vi "Init Tunnel References.vi"(8 "error in (no error)":errorcluster, 11 "CSM-Helper in":refnum<class "CSM-Helper.lvclass">) -> (0 "error out":errorcluster, 3 "CSM-Helper out":refnum<class "CSM-Helper.lvclass">)   [LabVIEW 2020, in "CSM-Helper.lvclass"]
uses:
  CSM-Helper.lvclass
  CSM-Helper.lvclass/CSM-Helper.ctl
  <vilib>/Utility/Data Type/Type Definitions/Data Type.ctl
  <vilib>/Utility/Data Type/Type Definitions/Refnum Type.ctl
  <vilib>/Utility/Data Type/NI_Data Type.lvlib
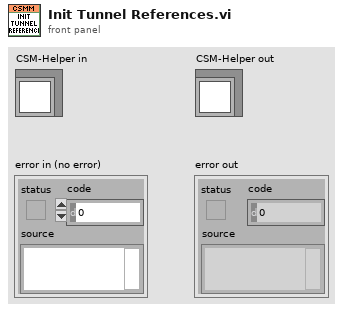
[diagram p1: front panel]
types:
  T1 = cluster{refnum<vi>, "Outer Term":refnum<vi>, "Data Type":variant, "Wire":refnum<vi>}
  T2 = typedef "NI_Data Type.lvlib/Data Type.ctl" = enum8{"Invalid Type", "Void", "I8", "I16", "I32", "I64", "U8", "U16", "U32", "U64", "Single Float", "Double Float", "Extended Float", "Single Complex", "Double Complex", "Extended Complex", "Enum U8", "Enum U16", "Enum U32", "Enum U64", "Single Float With Unit", "Double Float With Unit", "Extended Float With Unit", "Single Complex with Unit", "Double Complex with Unit", "Extended Complex with Unit", "Boolean", "String", "Path", "Picture", "Tag", "Array", "Cluster", "Variant", "LV Variant", "Waveform", "Timestamp", "Digital Waveform", "Digital Data", "ExpressData", "Refnum", "External Data", "VI", "Poly VI", "LabVIEW Class Instance", "Fixed Point", "Set Collection", "Map Collection"}
  T3 = typedef "NI_Data Type.lvlib/Type Definition Info.ctl" = cluster{"Name":string, "Timestamp":u32}
  T4 = typedef "NI_Data Type.lvlib/Refnum Type.ctl" = enum16{"NotARefnum", "UnknownRefnum", "Generic", "Datalog", "ByteStream", "Device", "Occurence", "TCPNetConnection", "Auto", "Menu", "Imaq", "Hardware", "DataSocket", "Visa", "IVI", "UDPNetConnection", "Notifier", "Queue", "Irda", "EventReg", "DotNet", "UserEvent", "Callback", "UNUSED_EMPTY_POSITION", "BlueToothNetConnection", "LVObjApp", "LVObjVI", "LVObjUnknown", "GenericClass", "UserDefinedRefnumTag", "DataValue", "RT FIFO", "TDMS File", "PythonSessionRefnum"}
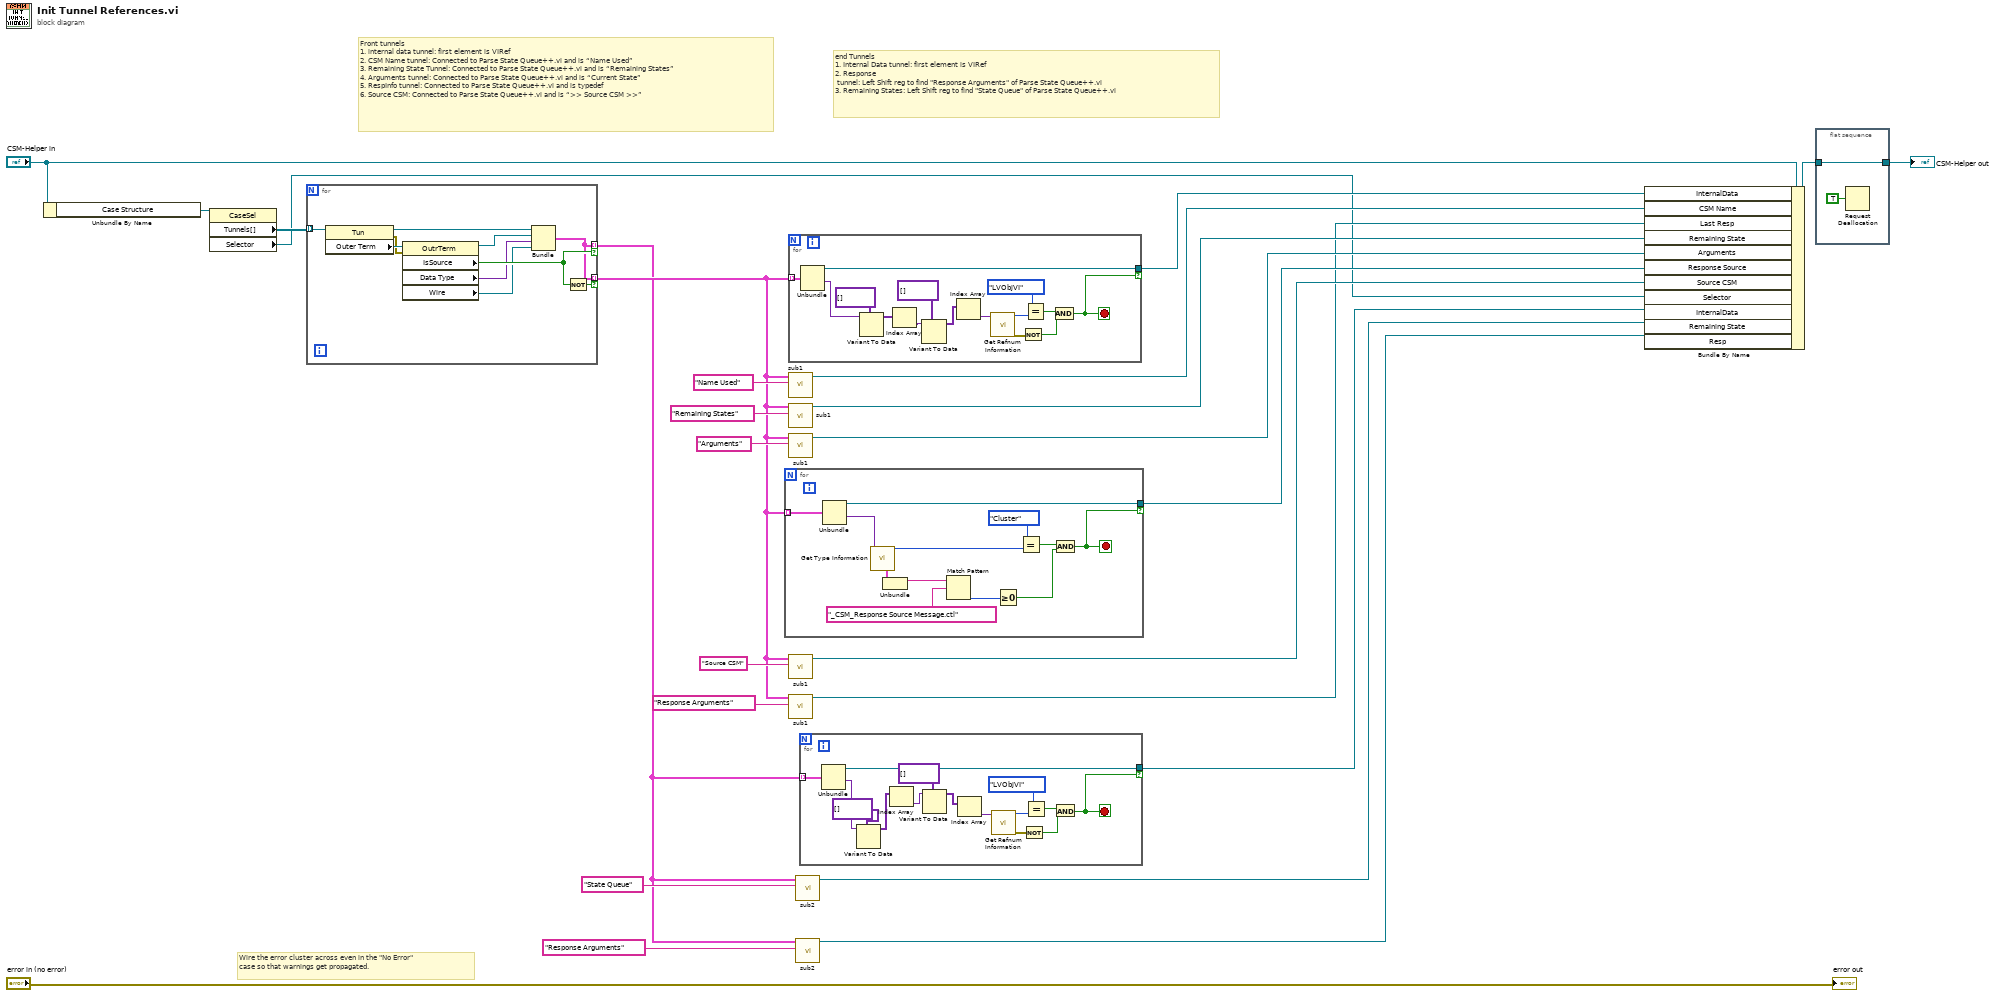
[diagram p0: block diagram]
diagram:
  # "end Tunnels\n1. Internal Data tunnel: first element is VIRef\n2. Response\n tunnel: Left Shift reg to find \"Response Arguments\" of Parse State Queue++.vi \n3. Remaining States: Left Shift reg to find \"State Queue\" of Parse State Queue++.vi"
  # "Front tunnels\n1. internal data tunnel: first element is VIRef\n2. CSM Name tunnel: Connected to Parse State Queue++.vi and is “Name Used”\n3. Remaining State Tunnel: Connected to Parse State Queue++.vi and is “Remaining States”\n4. Arguments tunnel: Connected to Parse State Queue++.vi and is “Current State”\n5. RespInfo tunnel: Connected to Parse State Queue++.vi and is typedef\n6. Source CSM: Connected to Parse State Queue++.vi and is “>> Source CSM >>”"
  # "Wire the error cluster across even in the \"No Error\"\ncase so that warnings get propagated."
  n1 = Unbundle By Name("CSM-Helper in") -> ("Case Structure"=w24:refnum<vi>)
  n2 = property class="CaseSel"(reference=w24) -> ("Tunnels[]"=w23:refnum<vi>[], "Selector"=w9:refnum<vi>)  [unwired: 1 in, 2 out]
  n3 = for {
    tunnel: w23 -> [w36] mode=indexing
    tunnel: [w29] -> w3 mode=indexing if=w33
    tunnel: [w29] -> w12 mode=indexing if=w32
    n4 = property class="Tun"(reference=w36) -> (reference out=w31:refnum<vi>, error out=w34:errorcluster, "Outer Term"=w35:refnum<vi>)  [unwired: 1 in]
    n5 = property class="OutrTerm"(reference=w35, error in=w34) -> (reference out=w30:refnum<vi>, "IsSource"=w33:bool, "Data Type"=w28:variant, "Wire"=w27:refnum<vi>)  [unwired: 1 out]
    n6 = Bundle(w31, "Outer Term"=w30, "Data Type"=w28, "Wire"=w27) -> (w29:T1)  [unwired: 1 in]
    n7 = Not(x=w33) -> (.not. x?=w32:bool)
  }
  n8 = for {
    tunnel: w12 -> [w48] mode=indexing
    tunnel: [w45] -> w13 if=w44
    stop <- w44 stop-if-true
    n9 = Unbundle(w48) -> (w45:refnum<vi>, "Data Type"=w41:variant)  [unwired: 2 out]
    n10 = call <vilib>:"Get Type Information.vi"("variant"=w41) -> ("type"=w47:T2, "type definition info"=w42:T3)  [unwired: 6 in, 3 out]
    n11 = Unbundle(w42) -> ("Name"=w40:string)  [unwired: 1 out]
    n12 = Match Pattern(string=w40, regular expression="_CSM_Response Source Message.ctl") -> (offset past match=w38:i32)  [unwired: 1 in, 3 out]
    n13 = Greater Or Equal To 0?(x=w38) -> (x >= 0?=w37:bool)
    n14 = Equal?(x=Data_Type."Cluster", y=w47) -> (x = y?=w46:bool)
    n15 = And(x=w46, y=w37) -> (x .and. y?=w44:bool)
  }
  n16 = for {
    tunnel: w12 -> [w63] mode=indexing
    tunnel: [w56] -> w22 if=w55
    stop <- w55 stop-if-true
    n17 = Unbundle(w63) -> (w56:refnum<vi>, "Data Type"=w53:variant)  [unwired: 2 out]
    n18 = Variant To Data(type=variant[] [] ("Array"), Variant=w53) -> (data=w52:variant[])  [unwired: 1 in, 1 out]
    n19 = Index Array(array=w52) -> (element=w50:variant)  [unwired: 1 in]
    n20 = Variant To Data(type=variant[] [] ("Array"), Variant=w50) -> (data=w49:variant[])  [unwired: 1 in, 1 out]
    n21 = Index Array(array=w49) -> (element=w62:variant)  [unwired: 1 in]
    n22 = call <vilib>:"Get Refnum Information.vi"("variant"=w62) -> ("error out"=w58:errorcluster, "reference type"=w60:T4)  [unwired: 7 in, 2 out]
    n23 = Not(x=w58) -> (.not. x?=w57:bool)
    n24 = Equal?(x=Refnum_Type."LVObjVI", y=w60) -> (x = y?=w59:bool)
    n25 = And(x=w59, y=w57) -> (x .and. y?=w55:bool)
  }
  n26 = call "sub1.vi"("regular expression"="Name Used", "Array"=w12) -> ("Tunnel out"=w21:refnum<vi>)  [unwired: 9 in]
  n27 = call "sub1.vi"("regular expression"="Remaining States", "Array"=w12) -> ("Tunnel out"=w18:refnum<vi>)  [unwired: 9 in]
  n28 = call "sub1.vi"("regular expression"="Arguments", "Array"=w12) -> ("Tunnel out"=w16:refnum<vi>)  [unwired: 9 in]
  n29 = call "sub1.vi"("regular expression"="Source CSM", "Array"=w12) -> ("Tunnel out"=w14:refnum<vi>)  [unwired: 9 in]
  n30 = call "sub1.vi"("regular expression"="Response Arguments", "Array"=w12) -> ("Tunnel out"=w10:refnum<vi>)  [unwired: 9 in]
  n31 = call "sub2.vi"("regular expression"="State Queue", "Array"=w3) -> ("Tunnel out"=w4:refnum<vi>)  [unwired: 9 in]
  n32 = call "sub2.vi"("regular expression"="Response Arguments", "Array"=w3) -> ("Tunnel out"=w1:refnum<vi>)  [unwired: 9 in]
  n33 = for {
    tunnel: w3 -> [w78] mode=indexing
    tunnel: [w71] -> w6 if=w70
    stop <- w70 stop-if-true
    n34 = Unbundle(w78) -> (w71:refnum<vi>, "Data Type"=w66:variant)  [unwired: 2 out]
    n35 = Variant To Data(type=variant[] [] ("Array"), Variant=w66) -> (data=w64:variant[])  [unwired: 1 in, 1 out]
    n36 = Index Array(array=w64) -> (element=w68:variant)  [unwired: 1 in]
    n37 = Variant To Data(type=variant[] [] ("Array"), Variant=w68) -> (data=w67:variant[])  [unwired: 1 in, 1 out]
    n38 = Index Array(array=w67) -> (element=w77:variant)  [unwired: 1 in]
    n39 = call <vilib>:"Get Refnum Information.vi"("variant"=w77) -> ("error out"=w73:errorcluster, "reference type"=w75:T4)  [unwired: 7 in, 2 out]
    n40 = Not(x=w73) -> (.not. x?=w72:bool)
    n41 = Equal?(x=Refnum_Type."LVObjVI", y=w75) -> (x = y?=w74:bool)
    n42 = And(x=w74, y=w72) -> (x .and. y?=w70:bool)
  }
  n43 = Bundle By Name(cluster="CSM-Helper in", "InternalData"=w22, "CSM Name"=w21, "Last Resp"=w10, "Remaining State"=w18, "Arguments"=w16, "Response Source"=w13, "Source CSM"=w14, "Selector"=w9, "InternalData"=w6, "Remaining State"=w4, "Resp"=w1) -> (w8:refnum<class "CSM-Helper.lvclass">)
  n44 = flat-sequence {
    tunnel: w8 -> [w79]
    tunnel: [w79] -> w7
    frame #0 {
      n45 = Request Deallocation(TRUE ("flag")) -> ()
    }
  }
  "error out" <- "error in (no error)"
  "CSM-Helper out" <- w7
